vi "Size Of.vi"(8 "错误输入（无错误）":errorcluster, 11 "Type":variant) -> (0 "错误输出":errorcluster, 3 "Bit Accurate Data Size For Type":u32)   [LabVIEW 2012, in "Application.lvlib"]
uses:
  Application.lvlib
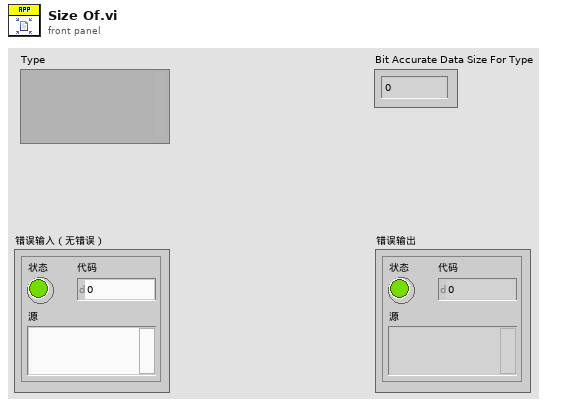
[diagram p1: front panel]
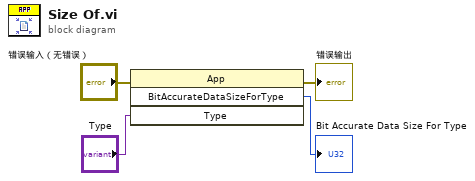
[diagram p0: block diagram]
diagram:
  n1 = invoke class="App" method="BitAccurateDataSizeForType"(error in="错误输入（无错误）", "Type"="Type") -> (error out=→"错误输出":errorcluster, "BitAccurateDataSizeForType"=→"Bit Accurate Data Size For Type":u32)  [unwired: 2 in, 2 out]
